vi "Create Status Log Header.vi"(8 "error in":errorcluster, 11 "Log File Refnum in":refnum<file>) -> (0 "error out":errorcluster, 3 "Log File Refnum out":refnum<file>)   [LabVIEW 2014]
uses:
  Boiler System Globals.vi
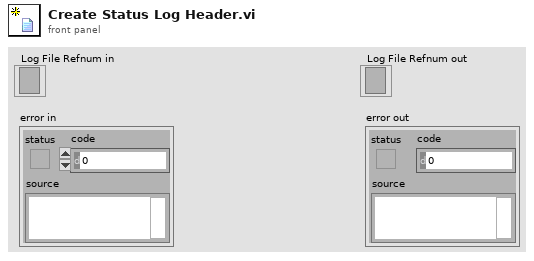
[diagram p1: front panel]
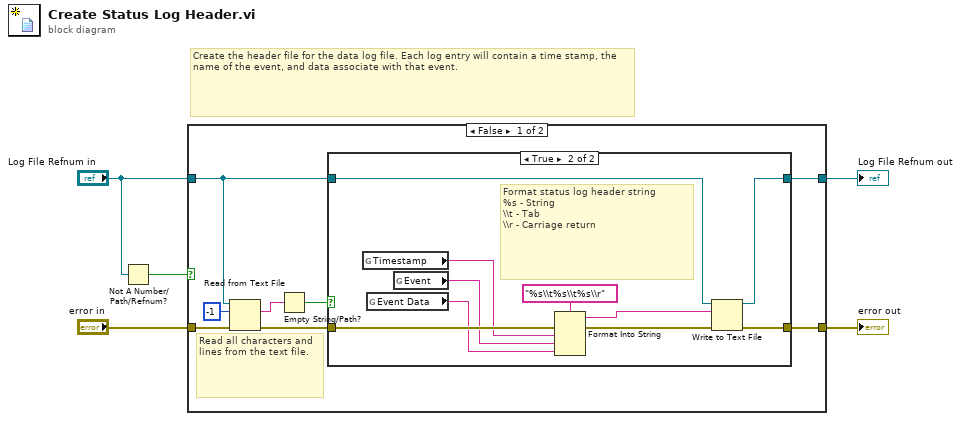
[diagram p0: block diagram]
diagram:
  # "Create the header file for the data log file. Each log entry will contain a time stamp, the name of the event, and data associate with that event."
  n1 = Not A Number/Path/Refnum?(number/path/refnum="Log File Refnum in") -> (NaN/Path/Refnum?=w1:bool)
  n2 = case shown="False" w1 {
    tunnel: [w11 w26] -> w5
    tunnel: [w10 w27] -> w4
    tunnel: "error in" -> [w7 w27]
    tunnel: "Log File Refnum in" -> [w6 w26]
    frame False {
      # "Read all characters and lines from the text file."
      n3 = Read from Text File(file (use dialog)=w6, count=-1, error in=w7) -> (text=w13:string, error out=w9:errorcluster)  [unwired: 1 in, 2 out]
      n4 = Empty String/Path?(string/path=w13) -> (empty?=w12:bool)
      n5 = case shown="True" w12 {
        tunnel: w9 -> [w15 w20]
        tunnel: w6 -> [w14 w25]
        tunnel: [w15 w24] -> w10
        tunnel: [w14 w23] -> w11
        frame False {
        }
        frame True {
          # "Format status log header string\n%s - String\n\\\\t - Tab\n\\\\r - Carriage return"
          n6 = global read "Boiler System Globals.vi" "Timestamp"() -> (w16:string)
          n7 = global read "Boiler System Globals.vi" "Event Data"() -> (w17:string)
          n8 = global read "Boiler System Globals.vi" "Event"() -> (w18:string)
          n9 = Format Into String(format string="%s\\t%s\\t%s\\r", error in=w20, w16, w18, w17) -> (resulting string=w22:string, error out=w21:errorcluster)  [unwired: 1 in]
          n10 = Write to Text File(file (use dialog)=w25, text=w22, error in=w21) -> (refnum out=w23:refnum<file>, error out=w24:errorcluster)  [unwired: 1 in, 1 out]
        }
      }
    }
    frame True {
    }
  }
  "Log File Refnum out" <- w5
  "error out" <- w4
